vi "Write Mensajes.vi"(8 "error in (no error)":errorcluster, 10 "Mensajes":refnum<user-event>, 11 "Monedas in":refnum<class "Monedas.lvclass">) -> (0 "error out":errorcluster, 3 "Monedas out":refnum<class "Monedas.lvclass">)   [LabVIEW 2020, in "Monedas.lvlib" / "Monedas.lvclass"]
uses:
  Monedas.lvclass
  Monedas.lvclass/Monedas.ctl
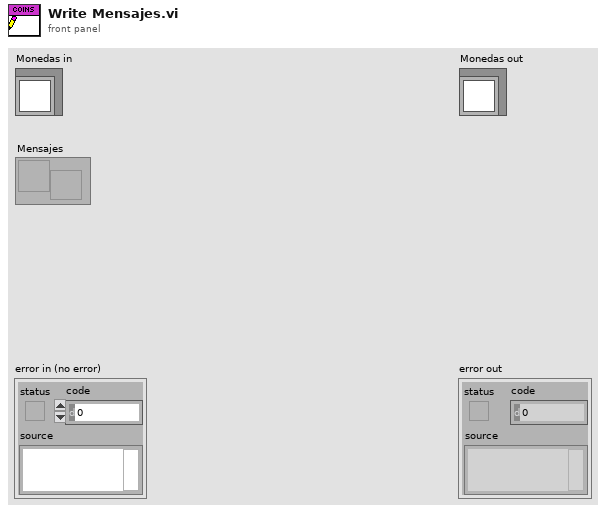
[diagram p1: front panel]
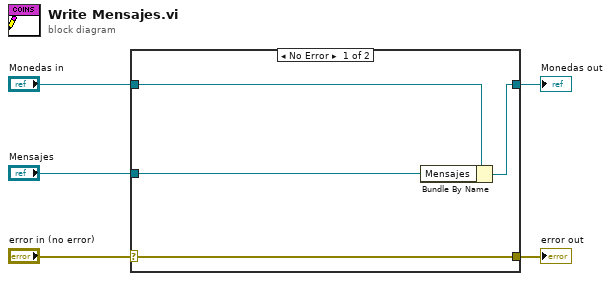
[diagram p0: block diagram]
diagram:
  n1 = case shown="No Error" "error in (no error)" {
    selector: "error in (no error)" -> [w9 w10]
    tunnel: [w9 w10] -> w4
    tunnel: [w7 w11] -> w2
    tunnel: "Monedas in" -> [w8 w11]
    tunnel: "Mensajes" -> [w6 _]
    frame No Error {
      n2 = Bundle By Name(cluster=w8, "Mensajes"=w6) -> (w7:refnum<class "Monedas.lvclass">)
    }
    frame Error {
    }
  }
  "error out" <- w4
  "Monedas out" <- w2
